vi "utils_GetSubVITerms.vi"(2 "Drop VI":bool, 3 "XRef":refnum<vi>, 4 "State In":T1, 5 "Path":path) -> (0 "Reply":string[](array[string]), 1 "State Out":T1)   [LabVIEW 2018, in "RetryNode.xnode"]
uses:
  RetryNode.xnode
  State.ctl
  <vilib>/Utility/miscctls.llb/LVRectTypeDef.ctl
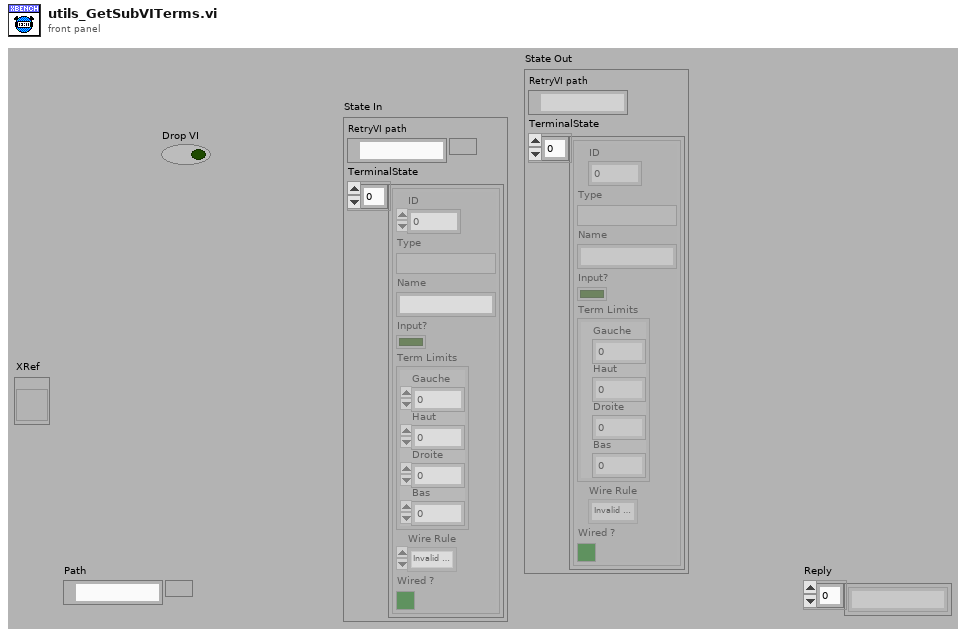
[diagram p1: front panel]
types:
  T1 = typedef "RetryNode.xnode/State.ctl" = cluster{"RetryVI path":path, "TerminalState":cluster{"ID":i32, "Type":variant, "Name":string, "Input?":bool, "Term Limits":T2, "Wire Rule":enum16{"Invalid Wire Rule", "Required", "Recommended", "Optional", "Dynamic Dispatch"}, "Wired ?":bool}[]}
  T2 = typedef "LVRectTypeDef.ctl" = cluster{"Left":i16, "Top":i16, "Right":i16, "Bottom":i16}
  T3 = cluster{"ID":i32, "Type":variant, "Name":string, "Input?":bool, "Term Limits":T2, "Wire Rule":enum16{"Invalid Wire Rule", "Required", "Recommended", "Optional", "Dynamic Dispatch"}, "Wired ?":bool}[]
  T4 = cluster{"ID":i32, "Type":variant, "Name":string, "Input?":bool, "Term Limits":T2, "Wire Rule":enum16{"Invalid Wire Rule", "Required", "Recommended", "Optional", "Dynamic Dispatch"}, "Wired ?":bool}
  T5 = enum16{"Invalid Wire Rule", "Required", "Recommended", "Optional", "Dynamic Dispatch"}[]
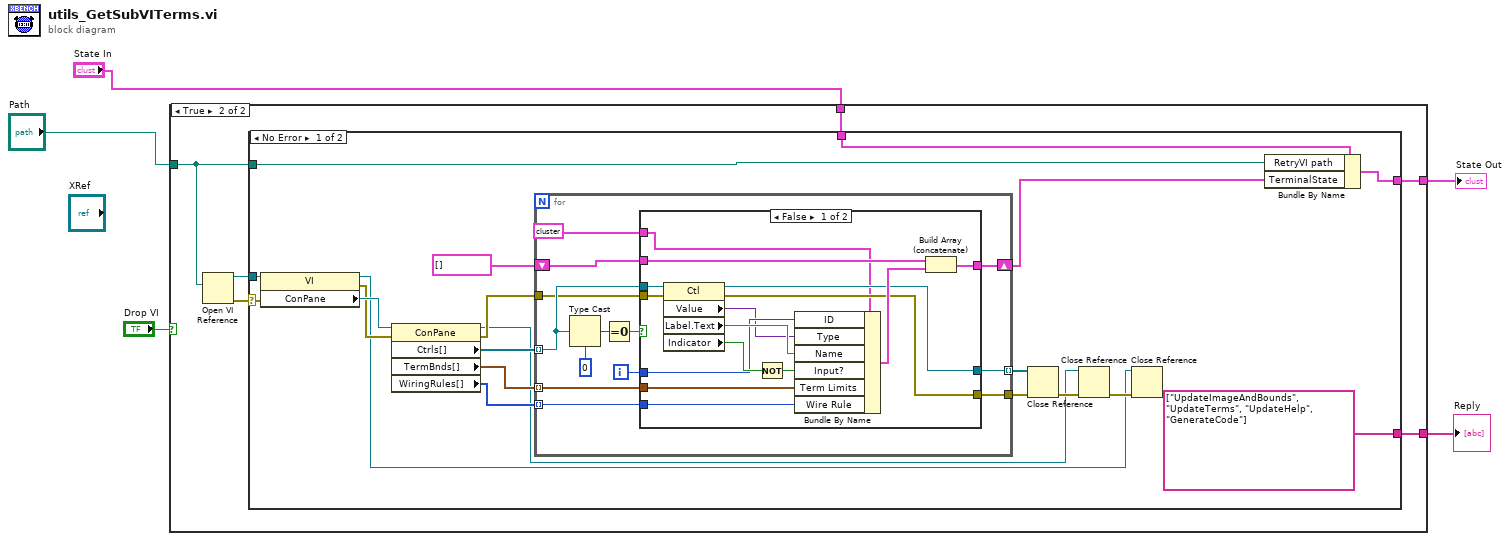
[diagram p0: block diagram]
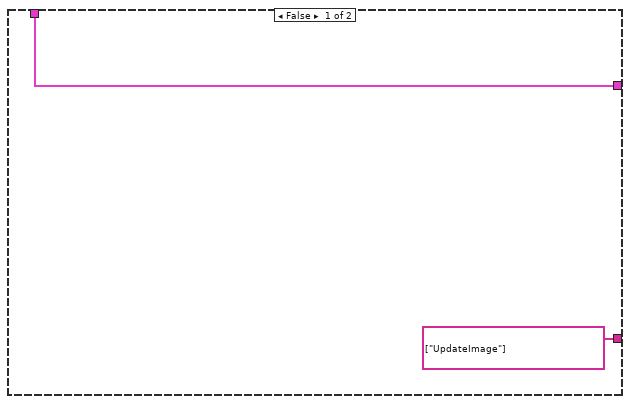
[diagram p2: hidden frame]
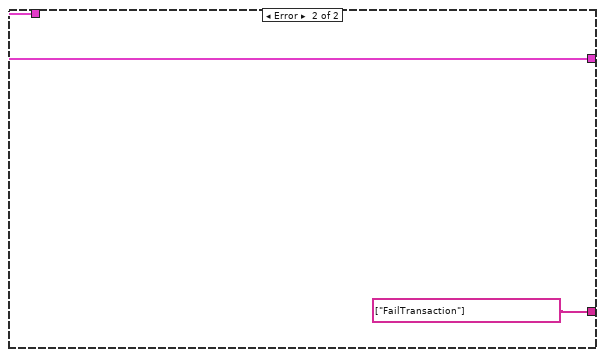
[diagram p4: hidden frame]
diagram:
  n1 = case shown="True" "Drop VI" {
    tunnel: [string[] ["UpdateImage"] ("Reply") w13] -> w5
    tunnel: "Path" -> [_ w12]
    tunnel: [w6 w11] -> w3
    tunnel: "State In" -> [w6 w10]
    frame False {
    }
    frame True {
      n2 = Open VI Reference(vi path=w12) -> (vi reference=w8:refnum<vi>, error out=w9:errorcluster)  [unwired: 5 in]
      n3 = case shown="No Error" w9 {
        selector: w9 -> [w26 _]
        tunnel: w10 -> [w30 w66]
        tunnel: [w33 w66] -> w11
        tunnel: [string[] ["UpdateImageAndBounds", "UpdateTerms", "UpdateHelp", "GenerateCode"] ("Reply") string[] ["FailTransaction"] ("Reply")] -> w13
        tunnel: w12 -> [w31 _]
        tunnel: w8 -> [w29 _]
        frame No Error {
          n4 = property class="VI"(reference=w29, error in=w26) -> (reference out=w14:refnum<vi>, error out=w21:errorcluster, "ConPane"=w28:refnum<vi>)
          n5 = property class="ConPane"(reference=w28, error in=w21) -> (reference out=w16:refnum<vi>, error out=w22:errorcluster, "Ctrls[]"=w27:refnum<vi>[], "TermBnds[]"=w24:T2[], "WiringRules[]"=w23:T5)
          n6 = for {
            tunnel: w27 -> [w44] mode=indexing
            shift-right: [w46] -> w20
            shift-left: T3 [] ("Size") -> [w45]
            tunnel: w24 -> [w40] mode=indexing
            tunnel: w23 -> [w39] mode=indexing
            tunnel: w22 -> [w38]
            tunnel: [w36] -> w19 mode=indexing
            tunnel: [w35] -> w18
            i -> [w37]
            n7 = Type Cast(type=0, x=w44) -> (*(type *) &x=w42:i32)
            n8 = Equal To 0?(x=w42) -> (x = 0?=w41:bool)
            n9 = case shown="False" w41 {
              tunnel: w44 -> [w61 w63]
              tunnel: [w56 w64] -> w46
              tunnel: w45 -> [w55 w64]
              tunnel: w37 -> [w54 _]
              tunnel: w40 -> [w52 _]
              tunnel: w39 -> [w51 _]
              tunnel: w38 -> [w50 w62]
              tunnel: [w49 w63] -> w36
              tunnel: [w48 w62] -> w35
              tunnel: T4 {"ID"=0, "Type"=variant, "Name"="", "Input?"=FALSE, "Term Limits"={"Left"=0, "Top"=0, "Right"=0, "Bottom"=0}, "Wire Rule"=enum."Invalid Wire Rule", "Wired ?"=FALSE} ("Pearl") -> [w47 _]
              frame False {
                n10 = property class="Ctl"(reference=w61, error in=w50) -> (reference out=w49:refnum<vi>, error out=w48:errorcluster, "Value"=w53:variant, "Label.Text"=w60:string, "Indicator"=w59:bool)
                n11 = Not(x=w59) -> (.not. x?=w58:bool)
                n12 = Bundle By Name(cluster=w47, "ID"=w54, "Type"=w53, "Name"=w60, "Input?"=w58, "Term Limits"=w52, "Wire Rule"=w51) -> (w57:T4)
                n13 = Build Array (concatenate)(w55, w57) -> (w56:T3)
              }
              frame True {
              }
            }
          }
          n14 = Close Reference(reference=w19, error in (no error)=w18) -> (error out=w17:errorcluster)
          n15 = Close Reference(reference=w16, error in (no error)=w17) -> (error out=w15:errorcluster)
          n16 = Close Reference(reference=w14, error in (no error)=w15) -> ()  [unwired: 1 out]
          n17 = Bundle By Name(cluster=w30, "RetryVI path"=w31, "TerminalState"=w20) -> (w33:T1)
        }
        frame Error {
        }
      }
    }
  }
  "Reply" <- w5
  "State Out" <- w3
